vi "classCreationEditor.vi"(8 "error in (no error)":errorcluster) -> (0 "error out":errorcluster, 2 "stopMechanismType":T1=enum."BooleanUE", 3 "classPath":path)   [LabVIEW 2023]
uses:
  stopMechanismType.ctl
  <vilib>/Utility/error.llb/Trim Whitespace One-Sided.vi
panel:
  in  "stopMechanism":T2(ring) caption="Tak Channel"
  out "warning":string
  in  "cancel":bool
  in  "create":bool
  in  "folder":path caption="Save class to..."
  in  "className":string caption="Class name"
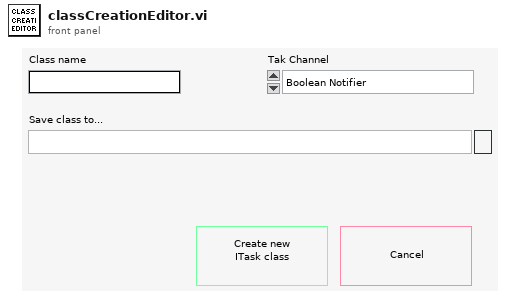
[diagram p1: front panel]
types:
  T1 = typedef "stopMechanismType.ctl" = enum16{"BooleanNotifier", "BooleanUE", "MsgUE"}
  T2 = enum16{"Boolean Notifier", "Boolean User Event", "Message User Event"}
  T3 = enum8{"Enabled", "Disabled", "Disabled and Grayed Out"}
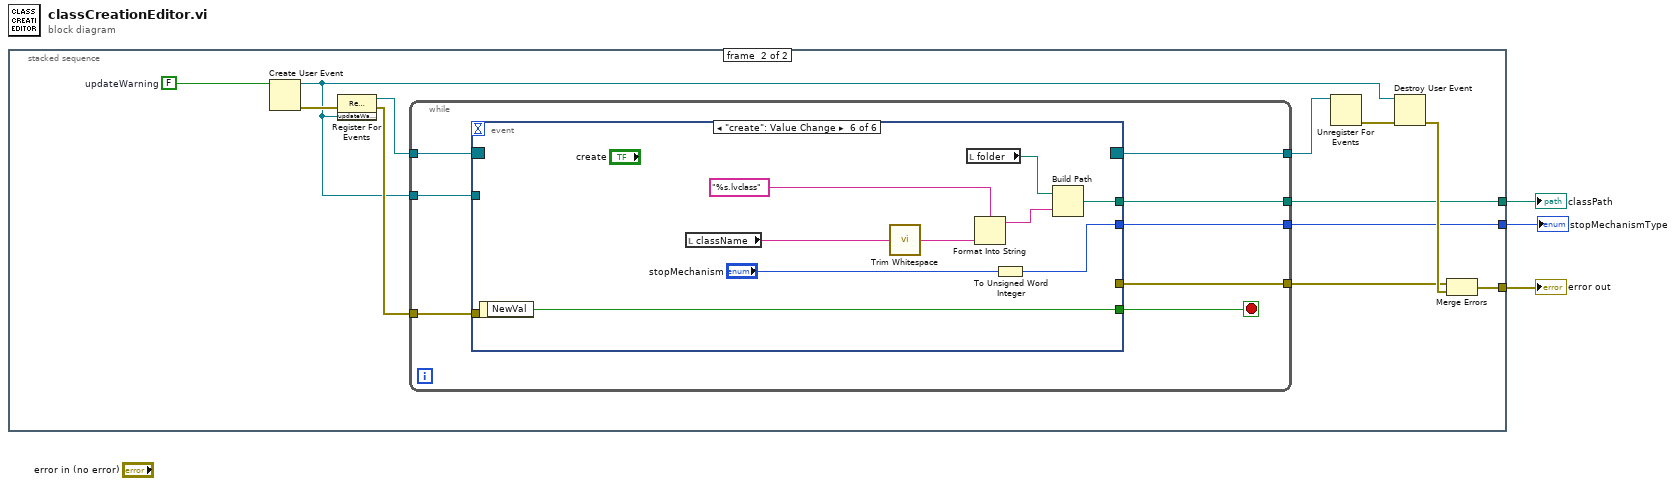
[diagram p0: block diagram]
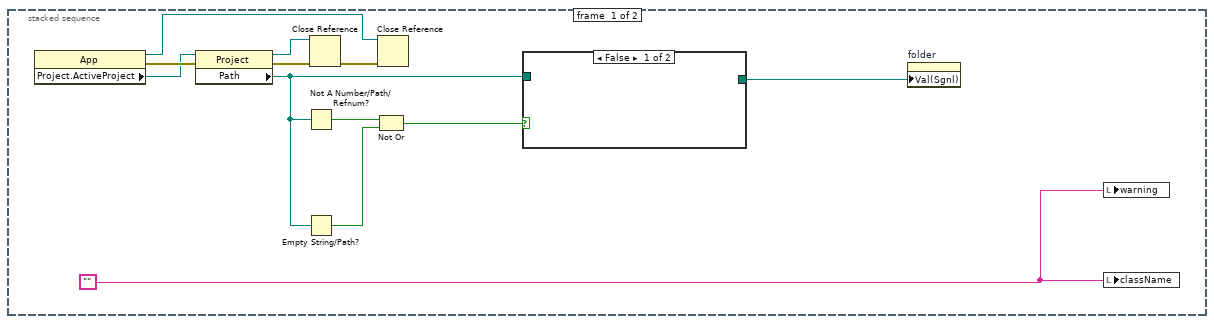
[diagram p2: hidden frame]
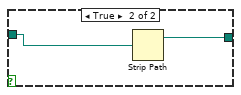
[diagram p3: hidden frame]
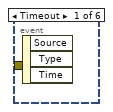
[diagram p4: hidden frame]
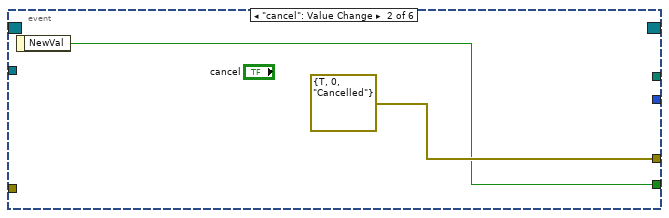
[diagram p5: hidden frame]
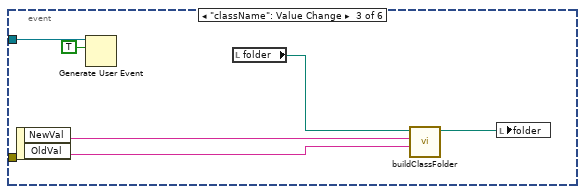
[diagram p6: hidden frame]
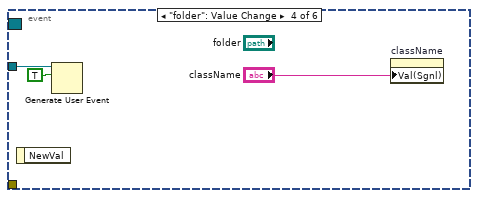
[diagram p7: hidden frame]
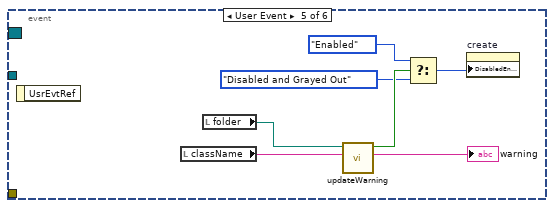
[diagram p8: hidden frame]
diagram:
  n1 = stacked-sequence {
    tunnel: [_ w21] -> w3
    tunnel: [_ w19] -> w2
    tunnel: [_ w18] -> w1
    frame #0 {
      w4 = ""
      n2 = property class="App"() -> (reference out=w15:refnum<vi>, error out=w13:errorcluster, "Project.ActiveProject"=w11:refnum<vi>)  [unwired: 2 in]
      n3 = property class="Project"(reference=w11, error in=w13) -> (reference out=w10:refnum<vi>, error out=w12:errorcluster, "Path"=w9:path)
      n4 = Not A Number/Path/Refnum?(number/path/refnum=w9) -> (NaN/Path/Refnum?=w7:bool)
      n5 = Empty String/Path?(string/path=w9) -> (empty?=w6:bool)
      n6 = Close Reference(reference=w10, error in (no error)=w12) -> (error out=w14:errorcluster)
      n7 = Not Or(1:w6, 2:w7) -> (0:w8:bool)
      n8 = Close Reference(reference=w15, error in (no error)=w14) -> ()  [unwired: 1 out]
      n9 = case shown="False" w8 {
        tunnel: w9 -> [_ w17]
        tunnel: [_ w16] -> w5
        frame False {
        }
        frame True {
          n10 = Strip Path(path=w17) -> (stripped path=w16:path)  [unwired: 1 out]
        }
      }
      n11 = property on="folder" class="Path"("Val(Sgnl)"=w5) -> ()  [unwired: 2 in, 2 out]
      n12 = local write "warning"(w4) -> ()
      n13 = local write "className"(w4) -> ()
    }
    frame #1 {
      w29 = FALSE  # updateWarning
      n14 = Create User Event(user event datatype=w29) -> (user event=w20:refnum<user-event>, error out=w25:errorcluster)  [unwired: 1 in]
      n15 = register-events(error in=w25, w20) -> (reference out=w28:refnum<event-registration>, error out=w24:errorcluster)  [unwired: 1 in]
      n16 = while {
        tunnel: [w37] -> w22
        tunnel: w28 -> [w35]
        tunnel: [w34] -> w27
        tunnel: w24 -> [w33]
        tunnel: w20 -> [w32]
        tunnel: [w31] -> w19
        tunnel: [w30] -> w18
        stop <- w36 stop-if-true
        n17 = event shown="[5] \"create\": Value Change" {
          selector: w35 -> [_ _ _ _ _ _]
          dyn-events: [_ _ _ _ _ _] -> w34
          timeout: _ -> [_ _ _ _ _ _]
          tunnel: [_ errorcluster {"status"=TRUE, "code"=0, "source"="Cancelled"} ("error out") _ _ _ _] -> w37
          tunnel: [_ w38 _ _ _ w64] -> w36
          tunnel: w33 -> [_ _ _ _ _ _]
          tunnel: w32 -> [_ _ w41 w46 _ _]
          tunnel: [_ _ _ _ _ w58] -> w31
          tunnel: [_ _ _ _ _ w56] -> w30
          event Timeout {
            n18 = event-data() -> ()  [unwired: 1 in, 3 out]
          }
          event "cancel": Value Change {
            n19 = event-data() -> ("NewVal"=w38:bool)  [unwired: 1 in]
          }
          event "className": Value Change {
            n20 = event-data() -> ("NewVal"=w45:string, "OldVal"=w43:string)  [unwired: 1 in]
            n21 = Generate User Event(user event=w41, event data cluster=TRUE ("event data")) -> ()  [unwired: 2 in, 2 out]
            n22 = local read "folder"() -> (w44:path)
            n23 = call "buildClassFolder.vi"("OldVal"=w43, "NewVal"=w45, "folder"=w44) -> ("appended path"=w42:path)  [unwired: 8 in]
            n24 = local write "folder"(w42) -> ()
          }
          event "folder": Value Change {
            n25 = event-data() -> ()  [unwired: 1 in, 1 out]
            n26 = Generate User Event(user event=w46, event data cluster=TRUE ("event data")) -> ()  [unwired: 2 in, 2 out]
            n27 = property on="className" class="Str"("Val(Sgnl)"="className") -> ()  [unwired: 2 in, 2 out]
          }
          event User Event {
            n28 = event-data() -> ()  [unwired: 1 in, 1 out]
            n29 = local read "className"() -> (w55:string)
            n30 = local read "folder"() -> (w54:path)
            n31 = call "updateWarning.vi"("className"=w55, "folder"=w54) -> ("warningText"=→"warning":string, "ok?"=w53:bool)  [unwired: 8 in]
            n32 = Select(t=T3."Enabled" ("Disabled"), s=w53, f=T3."Disabled and Grayed Out" ("Disabled")) -> (s? t:f=w50:T3)
            n33 = property on="create" class="Bool"("DisabledEnum"=w50) -> ()  [unwired: 2 in, 2 out]
          }
          event "create": Value Change {
            n34 = event-data() -> ("NewVal"=w64:bool)  [unwired: 1 in]
            n35 = local read "className"() -> (w63:string)
            n36 = call <vilib>:"Trim Whitespace.vi"("string"=w63) -> ("trimmed string"=w62:string)  [unwired: 1 in]
            n37 = local read "folder"() -> (w60:path)
            n38 = Format Into String(format string="%s.lvclass", w62) -> (resulting string=w59:string)  [unwired: 2 in, 1 out]
            n39 = To Unsigned Word Integer(number="stopMechanism") -> (unsigned 16bit integer=w56:u16)
            n40 = Build Path(base path=w60, name or relative path=w59) -> (appended path=w58:path)
          }
        }
      }
      n41 = Unregister For Events(event registration refnum=w27) -> (error out=w26:errorcluster)  [unwired: 1 in]
      n42 = Destroy User Event(user event=w20, error in=w26) -> (error out=w23:errorcluster)
      n43 = Merge Errors(w22, w23) -> (w21:errorcluster)
    }
  }
  "error out" <- w3
  "classPath" <- w2
  "stopMechanismType" <- w1
